vi "testConnect.vi"(8 "error in (no error)":errorcluster) -> (0 "error out":errorcluster)   [LabVIEW 2018]
doc: "Test the connection of LabVIEW. The command line should provide two arguments: (1) path to the SAL LabVIEW monitor, and (2) path to the LV Lib. If they are not provided or do not exist, the default files in the test data will be used."
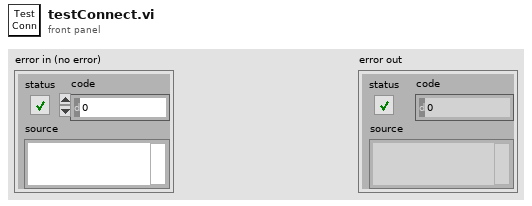
[diagram p1: front panel]
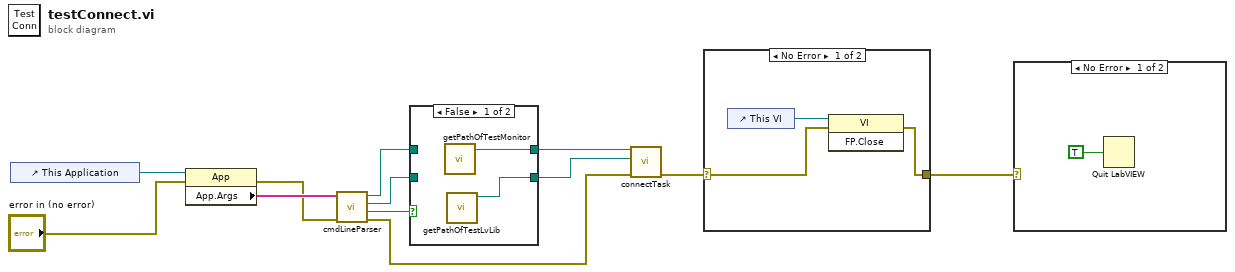
[diagram p0: block diagram]
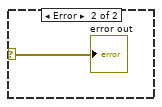
[diagram p2: hidden frame]
diagram:
  n1 = control-ref of="This Application"() -> (w12:refnum<vi>)
  n2 = property class="App"(reference=w12, error in="error in (no error)") -> (error out=w9:errorcluster, "App.Args"=w10:string[])  [unwired: 1 out]
  n3 = call "cmdLineParser.vi"("error in (no error)"=w9, "cmdLineArgs"=w10) -> ("error out"=w3:errorcluster, "filesExist"=w8:bool, "pathLvLib"=w6:path, "pathMonitor"=w7:path)  [unwired: 6 in]
  n4 = case shown="False" w8 {
    tunnel: w7 -> [_ w16]
    tunnel: w6 -> [_ w15]
    tunnel: [w14 w16] -> w5
    tunnel: [w13 w15] -> w4
    frame False {
      n5 = call "getPathOfTestMonitor.vi"() -> ("testMonitorPath"=w14:path)  [unwired: 11 in]
      n6 = call "getPathOfTestLvLib.vi"() -> ("testLvLibPath"=w13:path)  [unwired: 11 in]
    }
    frame True {
    }
  }
  n7 = call "connectTask.vi"("error in (no error)"=w3, "pathLvLib"=w4, "pathMonitor"=w5) -> ("error out"=w2:errorcluster)  [unwired: 8 in]
  n8 = case shown="No Error" w2 {
    selector: w2 -> [w17 w20]
    tunnel: [w18 w20] -> w1
    frame No Error {
      n9 = control-ref of="This VI"() -> (w19:refnum<vi>)
      n10 = invoke class="VI" method="FP.Close"(reference=w19, error in=w17) -> (error out=w18:errorcluster)  [unwired: 1 in, 2 out]
    }
    frame Error {
    }
  }
  n11 = case shown="No Error" w1 {
    selector: w1 -> [_ w22]
    frame No Error {
      n12 = Quit LabVIEW(quit? (T)=TRUE) -> ()
    }
    frame Error {
      "error out" <- w22
    }
  }
